vi "TrimBuffer.vi"(8 "error in (no error)":errorcluster, 11 "BufferedArray in":refnum<class "BufferedArray.lvclass">) -> (0 "error out":errorcluster, 3 "BufferedArray out":refnum<class "BufferedArray.lvclass">)   [LabVIEW 2017, in "LapDog.Collections.v0.Lists.Implementations.lvlib" / "BufferedArray.lvclass"]
doc: "Trim the tail half of the buffer. If the number of elements remaining after the trim is less than the minimum buffer size, only trim those elements above the minimum size limit."
uses:
  BufferedArray.lvclass
  BufferedArray.lvclass/BufferedArray.ctl
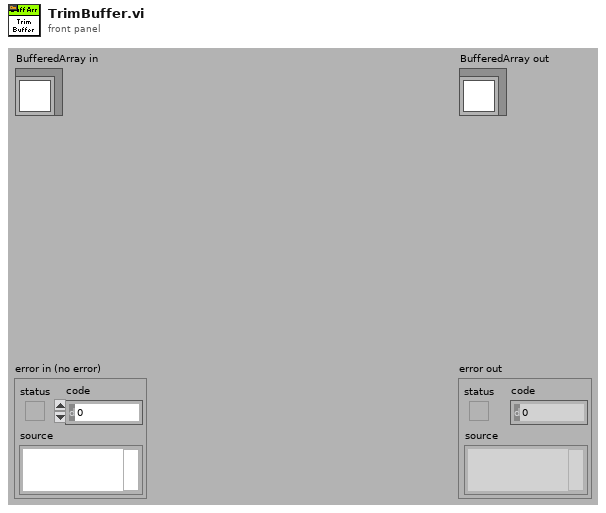
[diagram p1: front panel]
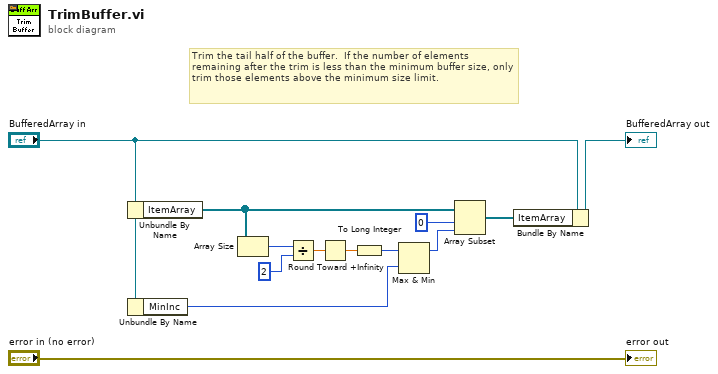
[diagram p0: block diagram]
diagram:
  # "Trim the tail half of the buffer.  If the number of elements remaining after the trim is less than the minimum buffer size, only trim those elements above the minimum size limit."
  n1 = Unbundle By Name("BufferedArray in") -> ("ItemArray"=w11:refnum<class>[])
  n2 = Unbundle By Name("BufferedArray in") -> ("MinInc"=w4:i32)
  n3 = Array Size(array=w11) -> (size(s)=w10:i32)
  n4 = Divide(x=w10, y=2) -> (x/y=w8:dbl)
  n5 = Round Toward +Infinity(x=w8) -> (ceil(x): smallest int >= x=w3:dbl)
  n6 = To Long Integer(number=w3) -> (32bit integer=w1:i32)
  n7 = Max & Min(x=w1, y=w4) -> (max(x,y)=w2:i32)  [unwired: 1 out]
  n8 = Array Subset(array=w11, index=0, length=w2) -> (w6:refnum<class>[])
  n9 = Bundle By Name(cluster="BufferedArray in", "ItemArray"=w6) -> (→"BufferedArray out":refnum<class "BufferedArray.lvclass">)
  "error out" <- "error in (no error)"
